vi "Set My Message.vi"(9 "ackNeeded":bool, 10 "args":variant, 11 "command":string) -> (3 "MyMessage":refnum<class "MyMessage.lvclass">)   [LabVIEW 2023, in "MyMessage.lvclass"]
uses:
  MyMessage.lvclass
  MyMessage.lvclass/MyMessage.ctl
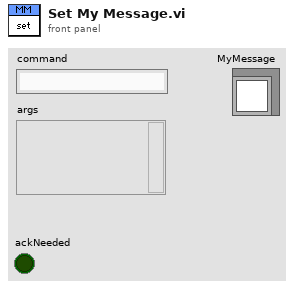
[diagram p1: front panel]
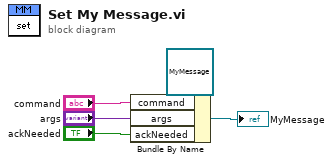
[diagram p0: block diagram]
diagram:
  n1 = Bundle By Name(cluster=refnum<class "MyMessage.lvclass"> refnum ("MyMessage.lvclass"), "command"="command", "args"="args", "ackNeeded"="ackNeeded") -> (→"MyMessage":refnum<class "MyMessage.lvclass">)
